vi "quickstart.vi"() -> ()   [LabVIEW 2013]
uses:
  IOTFoundation.lvlib
panel:
  in  "stop":bool
  out "Data Visualization":dbl(graph)
  in  "Credentials":T1={"Organization"="quickstart", "Device Type"="", "Device ID"="", "Auth token"=""}
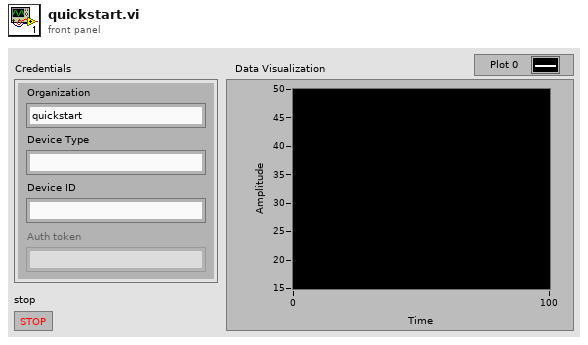
[diagram p1: front panel]
types:
  T1 = cluster{"Organization":string, "Device Type":string, "Device ID":string, "Auth token":string}
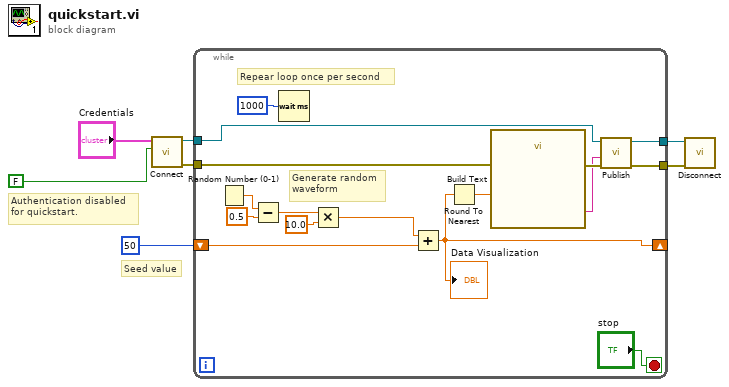
[diagram p0: block diagram]
diagram:
  # "Seed value"
  # "Authentication disabled\nfor quickstart."
  n1 = call "Connect.vi"("Credentials"="Credentials", "Authenticate"=FALSE) -> ("connection ID out"=w3:refnum<k5>, "error out"=w4:errorcluster)  [unwired: 5 in, 1 out]
  n2 = while {
    tunnel: w4 -> [w11]
    tunnel: [w13] -> w1
    tunnel: [w14] -> w2
    shift-right: [w15] -> _
    shift-left: 50 -> [w18]
    tunnel: w3 -> [w12]
    stop <- "stop" stop-if-true
    # "Repear loop once per second"
    # "Generate random\nwaveform"
    n3 = Random Number (0-1)() -> (number: 0 to 1=w23:dbl)
    n4 = Subtract(x=w23, y=0.5) -> (x-y=w21:dbl)
    n5 = Wait (ms)(milliseconds to wait=1000) -> ()  [unwired: 1 out]
    n6 = Multiply(x=w21, y=10.0) -> (x*y=w19:dbl)
    n7 = Add(x=w19, y=w18) -> (x+y=w15:dbl)
    "Data Visualization" <- w15
    n8 = Round To Nearest(number=w15) -> (nearest integer value=w8:dbl)
    n9 = call "Build Text"("rdm"=w8, "error in (no error)"=w11) -> ("Result"=w9:string, "error out"=w10:errorcluster)  [unwired: 12 in]
    n10 = call "Publish.vi"("error in (no error)"=w10, "Message to be published"=w9, "connection ID"=w12) -> ("error out"=w14:errorcluster, "connection ID out"=w13:refnum<k5>)  [unwired: 7 in]
  }
  n11 = call "Disconnect.vi"("error in (no error)"=w2, "connection ID"=w1) -> ()  [unwired: 9 in, 1 out]
